vi "Clear ALR_ACKs.vi"(8 "error in":errorcluster, 10 "N":i32, 11 "ALR_ON_OFF in":T1) -> (0 "error out":errorcluster, 3 "ALR_ON_OFF out":T1)   [LabVIEW 2019, in "Alarms.lvlib"]
uses:
  Alarms.lvlib
  Ctl/ALR_ON_OFF.ctl
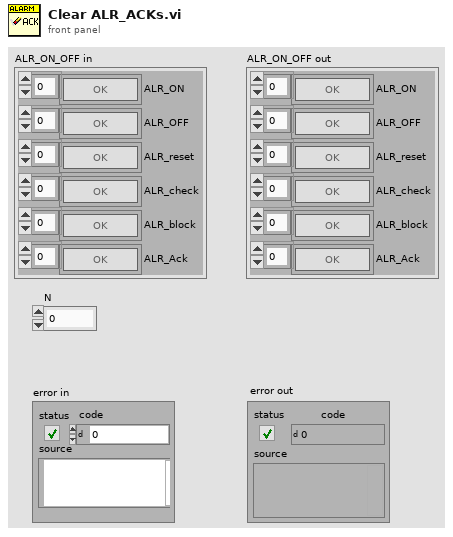
[diagram p1: front panel]
types:
  T1 = typedef "Alarms.lvlib/ALR_ON_OFF.ctl" = cluster{"ALR_ON":bool[], "ALR_OFF":bool[], "ALR_reset":bool[], "ALR_check":bool[], "ALR_block":bool[], "ALR_Ack":bool[]}
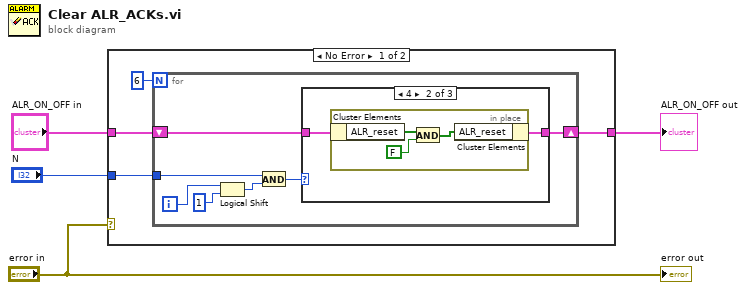
[diagram p0: block diagram]
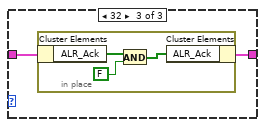
[diagram p3: hidden frame]
diagram:
  n1 = case shown="No Error" "error in" {
    tunnel: "N" -> [w8 _]
    tunnel: "ALR_ON_OFF in" -> [w7 w27]
    tunnel: [w6 w27] -> w3
    frame No Error {
      n2 = for {
        N: 6 -> [_]
        tunnel: w8 -> [w11]
        shift-right: [w9] -> w6
        shift-left: w7 -> [w13]
        i -> [w15]
        n3 = Logical Shift(y=w15, x=u8 1 ("y")) -> (x << y=w10:u8)
        n4 = And(x=w11, y=w10) -> (x .and. y?=w14:i32)
        n5 = case shown="4" w14 {
          tunnel: w13 -> [w16 w18 w23]
          tunnel: [w16 w17 w22] -> w9
          frame 0, Default {
          }
          frame 4 {
            n6 = in-place {
              n7 = in-place-cluster #1(w18) -> ("ALR_reset"=w21:bool[])
              n8 = And(x=w21, y=FALSE) -> (x .and. y?=w19:bool[])
              n9 = in-place-cluster #1("ALR_reset"=w19) -> (w17:T1)
            }
          }
          frame 32 {
            n10 = in-place {
              n11 = in-place-cluster #2(w23) -> ("ALR_Ack"=w26:bool[])
              n12 = And(x=w26, y=FALSE) -> (x .and. y?=w24:bool[])
              n13 = in-place-cluster #2("ALR_Ack"=w24) -> (w22:T1)
            }
          }
        }
      }
    }
    frame Error {
    }
  }
  "ALR_ON_OFF out" <- w3
  "error out" <- "error in"
